vi "testerVi.vi"() -> ()   [LabVIEW 2011, in "Hardware.lvlib" / "Channels.lvlib" / "niDAQmxAO.lvclass"]
uses:
  Channels/VoltOutput/niDAQmxAO.lvclass
  <vilib>/DAQmx/create/channels.llb/DAQmx Create Channel (AO-Voltage-Basic).vi
  Program Files/National Instruments/LabVIEW 2011/resource/objmgr/daqmx.rc
panel:
  out "DAQmx Task Name":refnum<k21>
  out "DAQmx Device Name":tag
  out "Channel Number":i32
  out "DAQmx Global Channel":refnum<k21>
  out "String":string
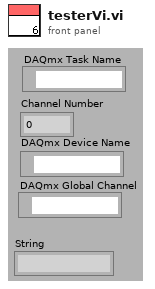
[diagram p1: front panel]
types:
  T1 = cluster{"Configuration Type":cluster{"Differential":i16, "Pseudodifferential":i16, "RSE":dbl}, "Voltage Type":cluster{"Voltage":string, "Current":string, "Standard Function ":cluster{"Sine":string, "Square":string, "Triangle":string}}}
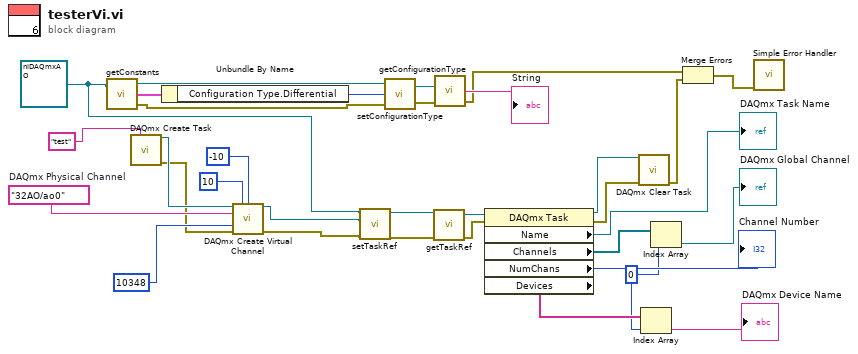
[diagram p0: block diagram]
diagram:
  w23 = 0
  w31 = tag "32AO/ao0"  # DAQmx Physical Channel
  w1 = refnum<class "niDAQmxAO.lvclass"> refnum ("Hardware:Channels.lvlib:niDAQmxAO.lvclass")
  n1 = call-dynamic "getConstants.vi"("niDAQmxAO.lvclass in"=w1) -> ("niDAQmxAO.lvclass out"=w6:refnum<class "niDAQmxAO.lvclass">, "Constants"=w33:T1, "error out"=w4:errorcluster)  [unwired: 1 in]
  n2 = call <vilib>:"DAQmx Create Task.vi"("new task name"="test") -> ("task out"=w18:refnum<k21>, "error out"=w16:errorcluster)  [unwired: 13 in]
  n3 = Unbundle By Name(w33) -> ("Configuration Type.Differential"=w5:i16)
  n4 = call-poly <vilib>:"DAQmx Create Virtual Channel.vi"("task in"=w18, "maximum value"=10, "minimum value"=-10, "physical channels"=w31, "units"=10348, "error in"=w16) -> ("task out"=w12:refnum<k21>, "error out"=w11:errorcluster)  [unwired: 8 in]
  n5 = call "setTaskRef.vi"("error in (no error)"=w11, "DAQmx Task Ref"=w12, "niDAQmxAO.lvclass in"=w1) -> ("error out"=w9:errorcluster, "niDAQmxAO.lvclass out"=w10:refnum<class "niDAQmxAO.lvclass">)  [unwired: 7 in]
  n6 = call "setConfigurationType.vi"("error in (no error)"=w4, "Configuration Type"=w5, "niDAQmxAO in"=w6) -> ("error out"=w3:errorcluster, "niDAQmxAO out"=w2:refnum<class "niDAQmxAO.lvclass">)
  n7 = call "getTaskRef.vi"("error in (no error)"=w9, "niDAQmxAO.lvclass in"=w10) -> ("error out"=w7:errorcluster, "DAQmx Task Ref"=w8:refnum<k21>)  [unwired: 7 in, 1 out]
  n8 = call "getConfigurationType.vi"("niDAQmxAO in"=w2, "error in (no error)"=w3) -> ("Configuration Type"=→"String":string, "error out"=w14:errorcluster)  [unwired: 1 out]
  n9 = property class="DAQmx Task"(reference=w8, error in=w7) -> (reference out=w20:refnum<k21>, error out=w19:errorcluster, "Name"=→"DAQmx Task Name":refnum<k21>, "Channels"=w27:refnum<k21>[], "NumChans"=→"Channel Number":u32, "Devices"=w24:tag[])
  n10 = call <vilib>:"DAQmx Clear Task.vi"("task in"=w20, "error in"=w19) -> ("error out"=w15:errorcluster)  [unwired: 13 in]
  n11 = Index Array(array=w24, index=w23) -> (element=→"DAQmx Device Name":tag)
  n12 = Index Array(array=w27, index=w23) -> (element=→"DAQmx Global Channel":refnum<k21>)
  n13 = Merge Errors(w14, w15) -> (w13:errorcluster)
  n14 = call <vilib>:"Simple Error Handler.vi"("error in (no error)"=w13) -> ()  [unwired: 4 in, 5 out]
